vi "test-CoerseNumericTypeFixedPoint.vi"() -> (0 "error out":errorcluster[](array[cluster]))   [LabVIEW 2019]
panel:
  out "x = y?":bool
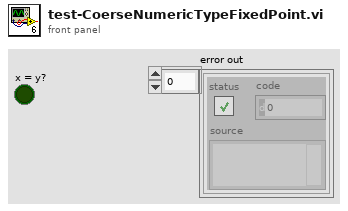
[diagram p1: front panel]
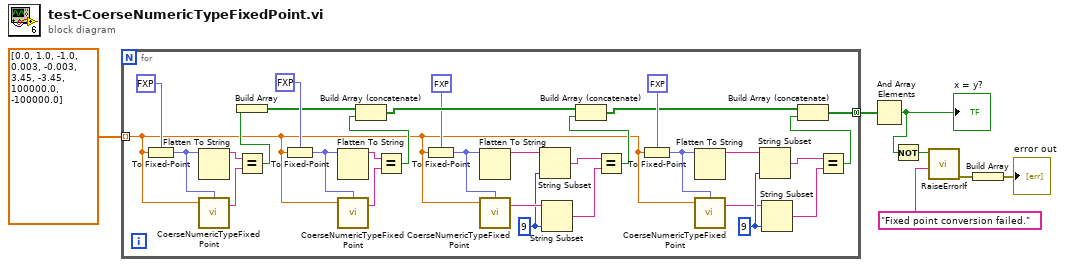
[diagram p0: block diagram]
diagram:
  n1 = for {
    tunnel: dbl[] [0.0, 1.0, -1.0, 0.003, -0.003, 3.45, -3.45, 100000.0, -100000.0] -> [w20] mode=indexing
    tunnel: [w18] -> w6 mode=concatenating
    w12 = 9 ("length (rest)")
    w13 = 9 ("length (rest)")
    n2 = To Fixed-Point(fixed-point type=fxp<+,16,8> 0.0, number=w20) -> (fixed-point=w35:fxp<+,16,8>)
    n3 = Flatten To String(anything=w35) -> (data string=w37:string)  [unwired: 3 in, 2 out]
    n4 = call "CoerseNumericTypeFixedPoint.vi"("Numeric Variant in"=w35, "Numeric"=w20) -> ("Encoded"=w36:string)  [unwired: 3 in]
    n5 = Equal?(x=w37, y=w36) -> (x = y?=w30:bool)
    n6 = Build Array(w30) -> (w29:bool[])
    n7 = To Fixed-Point(fixed-point type=fxp<+/-,16,8> 0.0, number=w20) -> (fixed-point=w34:fxp<+/-,16,8>)
    n8 = Flatten To String(anything=w34) -> (data string=w32:string)  [unwired: 3 in, 2 out]
    n9 = call "CoerseNumericTypeFixedPoint.vi"("Numeric Variant in"=w34, "Numeric"=w20) -> ("Encoded"=w33:string)  [unwired: 3 in]
    n10 = Equal?(x=w32, y=w33) -> (x = y?=w28:bool)
    n11 = Build Array (concatenate)(w29, w28) -> (w25:bool[])
    n12 = To Fixed-Point(fixed-point type=fxp<+,16,8> data[17B], number=w20) -> (fixed-point=w26:fxp<+,16,8>)
    n13 = Flatten To String(anything=w26) -> (data string=w17:string)  [unwired: 3 in, 2 out]
    n14 = call "CoerseNumericTypeFixedPoint.vi"("Numeric Variant in"=w26, "Numeric"=w20) -> ("Encoded"=w15:string)  [unwired: 3 in]
    n15 = String Subset(string=w17, length (rest)=w13) -> (substring=w16:string)  [unwired: 1 in]
    n16 = String Subset(string=w15, length (rest)=w13) -> (substring=w14:string)  [unwired: 1 in]
    n17 = Equal?(x=w16, y=w14) -> (x = y?=w27:bool)
    n18 = Build Array (concatenate)(w25, w27) -> (w19:bool[])
    n19 = To Fixed-Point(fixed-point type=fxp<+/-,16,8> data[17B], number=w20) -> (fixed-point=w22:fxp<+/-,16,8>)
    n20 = Flatten To String(anything=w22) -> (data string=w11:string)  [unwired: 3 in, 2 out]
    n21 = call "CoerseNumericTypeFixedPoint.vi"("Numeric Variant in"=w22, "Numeric"=w20) -> ("Encoded"=w10:string)  [unwired: 3 in]
    n22 = String Subset(string=w11, length (rest)=w12) -> (substring=w8:string)  [unwired: 1 in]
    n23 = String Subset(string=w10, length (rest)=w12) -> (substring=w9:string)  [unwired: 1 in]
    n24 = Equal?(x=w8, y=w9) -> (x = y?=w21:bool)
    n25 = Build Array (concatenate)(w19, w21) -> (w18:bool[])
  }
  n26 = And Array Elements(Boolean array=w6) -> (logical AND=w5:bool)
  "x = y?" <- w5
  n27 = Not(x=w5) -> (.not. x?=w4:bool)
  n28 = call "RaiseErrorIf.vi"("error message"="Fixed point conversion failed.", "error? (true)"=w4) -> ("error out"=w2:errorcluster)  [unwired: 9 in]
  n29 = Build Array(w2) -> (→"error out":errorcluster[])
